vi "lv-installer-build.vi"() -> (0 "error out":errorcluster)   [LabVIEW 2014, in "veristand-steps-build-system.lvlib"]
uses:
  <vilib>/Utility/error.llb/DialogType.ctl
  <vilib>/AppBuilder/AB_API_Simple/Build (path).vi
  veristand-steps-build-system.lvlib
  <vilib>/Wiresmith Technology/LabVIEW CLI/CLI Class/CLI.lvclass
  <vilib>/AppBuilder/AB_API_Simple/NI_App_Builder_API.lvlib
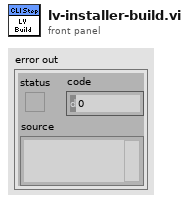
[diagram p1: front panel]
types:
  T1 = typedef "DialogType.ctl" = u16
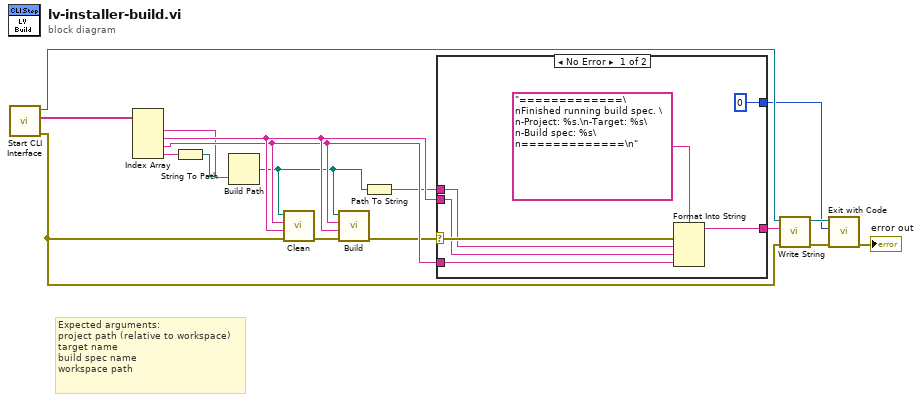
[diagram p0: block diagram]
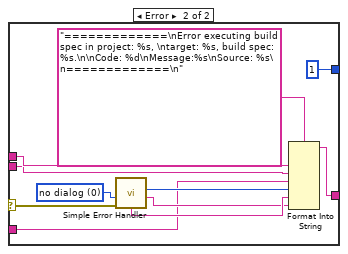
[diagram p2: hidden frame]
diagram:
  # "Expected arguments:\nproject path (relative to workspace)\ntarget name\nbuild spec name\nworkspace path"
  n1 = call <vilib>:"Start CLI Interface.vi"() -> ("error out"=w7:errorcluster, "Custom Parameters"=w17:string[], "CLI out"=w15:refnum<class "CLI.lvclass">)  [unwired: 9 in]
  n2 = Index Array(array=w17) -> (element #1=w6:string, element #2=w9:string, element #3=w8:string, element #4=w1:string)  [unwired: 4 in]
  n3 = String To Path(string=w1) -> (path=w2:path)
  n4 = Build Path(base path=w2, name or relative path=w6) -> (appended path=w4:path)
  n5 = call <vilib>:"Clean.vi"("error in (no error)"=w7, "Name of target (My Computer)"=w9, "Name of build specification (if empty: clean all)"=w8, "Path to project"=w4) -> ("error out"=w10:errorcluster)  [unwired: 7 in]
  n6 = call-poly <vilib>:"Build.vi"("error in (no error)"=w10, "Name of target (My Computer)"=w9, "Name of build specification (if empty: build all)"=w8, "Path to project"=w4) -> ("error out"=w5:errorcluster)  [unwired: 6 in, 1 out]
  n7 = Path To String(path=w4) -> (string=w3:string)
  n8 = case shown="No Error" w5 {
    selector: w5 -> [w23 w34]
    tunnel: w3 -> [w22 w27]
    tunnel: w9 -> [w21 w26]
    tunnel: [w20 w35] -> w16
    tunnel: [0 ("Exit Code (0)") 1 ("Exit Code (0)")] -> w12
    tunnel: w8 -> [w18 w25]
    frame No Error {
      n9 = Format Into String(format string="=============\nFinished running build spec. \n-Project: %s.\n-Target: %s\n-Build spec: %s\n=============\n", error in=w23, w22, w21, w18) -> (resulting string=w20:string)  [unwired: 1 in, 1 out]
    }
    frame Error {
      w33 = T1 0 items=["no dialog", "OK message", "continue or stop message", "OK message + warnings", "continue/stop + warnings"] ("type of dialog (OK msg:1)")
      n10 = call <vilib>:"Simple Error Handler.vi"("type of dialog (OK msg:1)"=w33, "error in (no error)"=w34) -> ("code out"=w28:i32, "source out"=w29:string, "message"=w30:string)  [unwired: 3 in, 2 out]
      n11 = Format Into String(format string="=============\nError executing build spec in project: %s, \ntarget: %s, build spec: %s.\n\nCode: %d\nMessage:%s\nSource: %s\n=============\n", w27, w26, w25, w28, w30, w29) -> (resulting string=w35:string)  [unwired: 2 in, 1 out]
    }
  }
  n12 = call <vilib>:"Write String.vi"("error in (no error)"=w7, "Text to Write"=w16, "CLI in"=w15) -> ("error out"=w14:errorcluster, "CLI out"=w13:refnum<class "CLI.lvclass">)  [unwired: 7 in]
  n13 = call <vilib>:"Exit with Code.vi"("error in (no error)"=w14, "Exit Code (0)"=w12, "CLI in"=w13) -> ("error out"=→"error out":errorcluster)  [unwired: 8 in]
